vi "PIDAutoTune_OpenLoop_ChooseMethod.vi"(4 "Sampling Time dt (s)":dbl, 5 "Constant Type":T2(ring), 6 "Kn":dbl, 7 "Type of Controller":u16(ring) items=["P", "PI", "PID"], 8 "Tune":bool, 9 "CO Offset":dbl=0.25, 10 "Measurement  (PV)":dbl, 11 "Control Output (Co)":dbl) -> (0 "Plant and Test Data":T3, 1 "New Tuning Parameters":T1, 2 "Tuning Done":bool, 3 "Adj CO":dbl)   [LabVIEW 2019, in "Trajectory_Library.lvlib"]
uses:
  Timer_New.vi
  LinearFilter_ResetToValue.vi
  LinearFilter_Calculate.vi
  <vilib>/Utility/semaphor.llb/Obtain Semaphore Reference.vi
  Timer_Reset.vi
  Timer_Start.vi
  Timer_Stop.vi
  Timer_HasPeriodPassedOnce.vi
  <vilib>/addons/control/pid/autopid.llb/PID Autotuning Design (Auto).vi
  <vilib>/addons/control/pid/autopid.llb/PID Autotuning Design (Chien-Hrones-Reswick).vi
  <vilib>/Analysis/Matrix/Numeric/Conversions/Array To Matrix - RA.vi
  LinearFilter_MovingAverage.vi
  LinearFilter_LowPassBW1.vi
  LinearFilter_LowPassBW2.vi
  LinearFilter_HighPassBW1.vi
  LinearFilter_HighPassBW2.vi
  Trajectory_Library.lvlib
  <vilib>/addons/control/pid/NI_PID_autopid.lvlib
  <vilib>/ptbypt/NI_PtbyPt.lvlib
  <vilib>/Analysis/Matrix/NI_Matrix.lvlib
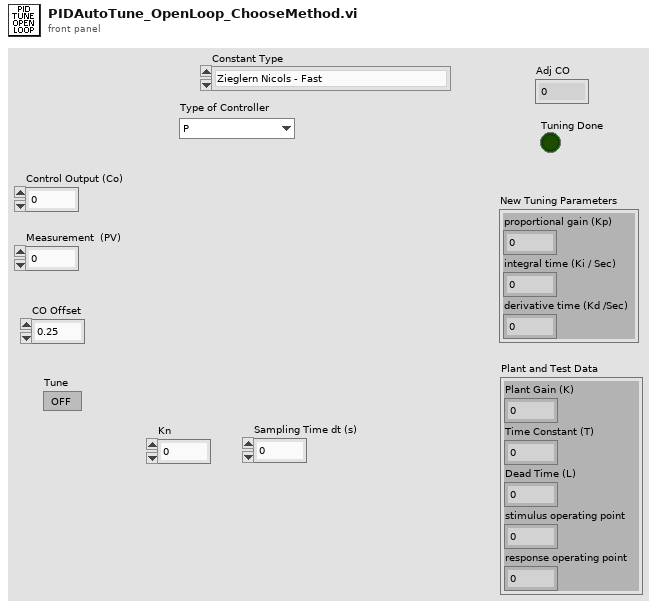
[diagram p1: front panel]
types:
  T1 = cluster{"proportional gain (Kp)":dbl, "integral time (Ki / Sec)":dbl, "derivative time (Kd /Sec)":dbl}
  T2 = enum16{"Zieglern Nicols - Fast", "Ziegler Nicols - Normal", "Ziegler Nicols - Slow", "CHR regulator - 0% overshoot", "CHR regulator - 20% overshoot", "CHR servo - 0 % overshoot", "CHR servo - 20% overshoot"}
  T3 = cluster{"Plant Gain (K)":dbl, "Time Constant (T)":dbl, "Dead Time (L)":dbl, "stimulus operating point":dbl, "response operating point":dbl}
  T4 = enum16{"Moving Average", "Low Pass 1st Order Butterworth", "Low Pass 2nd Order Butterworth", "High Pass 1st Order Butterworth", "High Pass 2nd Order Butterworth"}
  T5 = cluster{"proportional gain (Kc)":dbl, "integral time (Ti, min)":dbl, "derivative time (Td, min)":dbl}
  T6 = cluster{"Plant Gain (K)":dbl, "Time Constant (T)":dbl, "Dead Time (L)":dbl}
  T7 = typedef "NI_Matrix.lvlib/RealMatrix.ctl" = dbl[][]
  T8 = cluster{"Plant Gain (K)":dbl, "Time Constant (T)":dbl, "Dead Time (L)":dbl, "stimulus offset":dbl, "response offset":dbl}
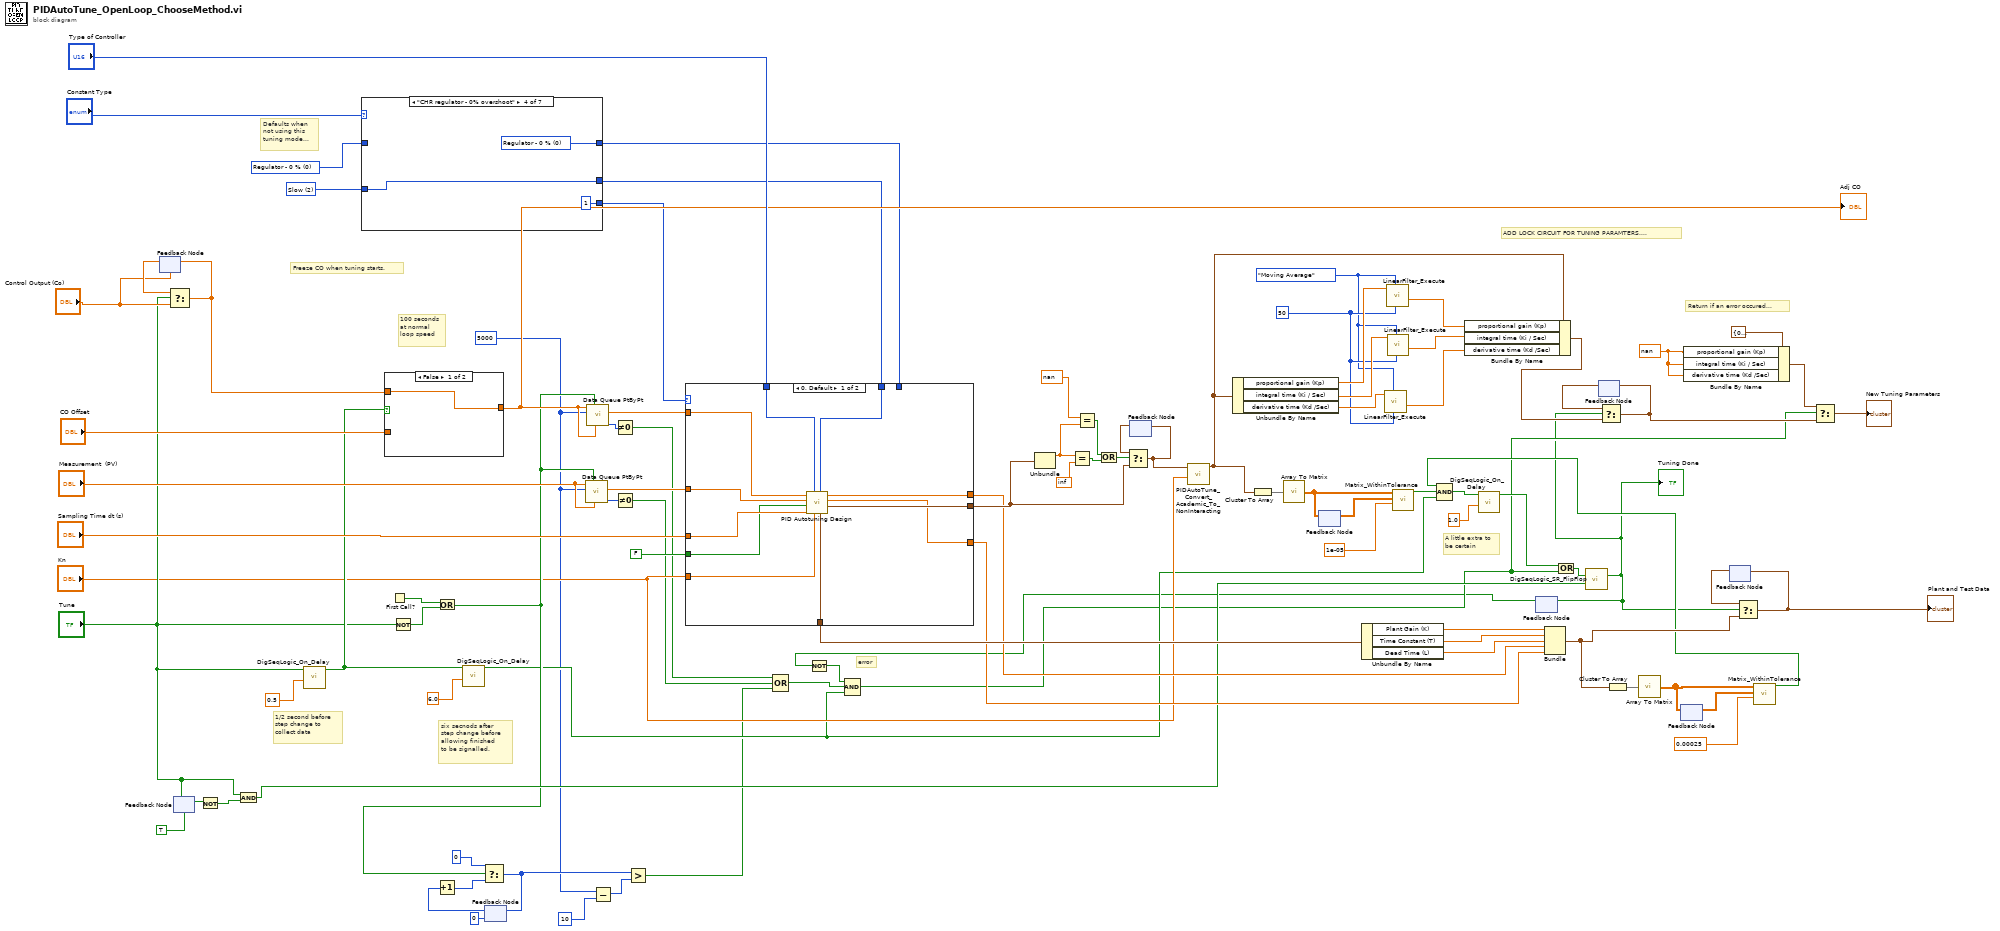
[diagram p0: block diagram]
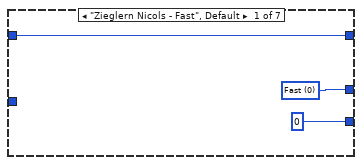
[diagram p2: hidden frame]
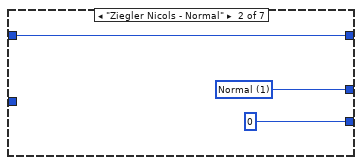
[diagram p3: hidden frame]
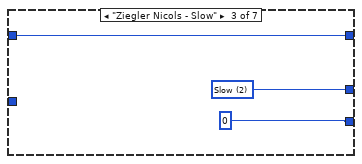
[diagram p4: hidden frame]
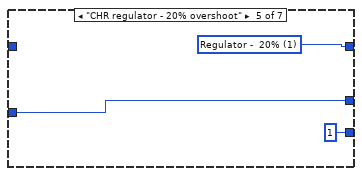
[diagram p5: hidden frame]
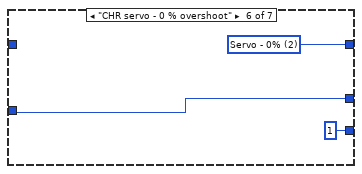
[diagram p6: hidden frame]
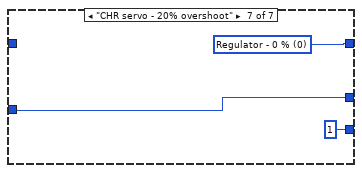
[diagram p7: hidden frame]
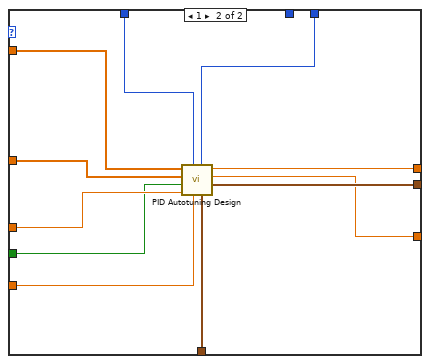
[diagram p8: hidden frame]
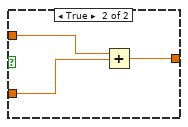
[diagram p9: hidden frame]
diagram:
  w22 = nan
  w50 = 50 ("Samples")
  w49 = T4."Moving Average" ("Filter Type")
  w55 = u16 2 items=["Fast", "Normal", "Slow"] ("Ziegler-Nichols Speed")
  w56 = u16 0 items=["Regulator - 0 %", "Regulator -  20%", "Servo - 0%", "Servo - 20%"] ("Tuning specifications")
  w8 = 5000 ("sample length")
  # "error"
  # "Return if an error occured..."
  # "A little extra to\nbe certain"
  # "Defaults when\nnot using this\ntuning mode..."
  # "100 seconds\nat normal\nloop speed"
  # "Freeze CO when tuning starts."
  # "ADD LOCK CIRCUIT FOR TUNING PARAMTERS...."
  # "six secnods after\nstep change before\nallowing finished \nto be signalled."
  # "1/2 second before\nstep change to\ncollect data"
  n1 = feedback #1("Control Output (Co)") -> (w73:dbl)
  n2 = Select(t=w73, s="Tune", f="Control Output (Co)") -> (s? t:f=w74:dbl)
  n3 = feedback-in #1(w74) -> ()
  n4 = feedback-in #2("Tune") -> ()
  n5 = feedback #2(TRUE ("Tune")) -> (w69:bool)
  n6 = Not(x=w69) -> (.not. x?=w67:bool)
  n7 = And(x="Tune", y=w67) -> (x .and. y?=w66:bool)
  n8 = call "DigSeqLogic_On_Delay.vi"("Delay"=0.5, "Input"="Tune") -> ("Output"=w76:bool)  [unwired: 8 in, 1 out]
  n9 = case shown="\"CHR regulator - 0% overshoot\"" "Constant Type" {
    tunnel: [w99 w102 w105 w106 w109 w112 w115] -> w59
    tunnel: [0 0 0 1 1 1 1] -> w58
    tunnel: [w97 w100 w103 w107 w110 w113 w116] -> w57
    tunnel: w56 -> [w97 w100 w103 _ _ _ _]
    tunnel: w55 -> [_ _ _ w106 w109 w112 w115]
    frame "Zieglern Nicols - Fast", Default {
      w99 = u16 0 items=["Fast", "Normal", "Slow"] ("Ziegler-Nichols Speed")
    }
    frame "Ziegler Nicols - Normal" {
      w102 = u16 1 items=["Fast", "Normal", "Slow"] ("Ziegler-Nichols Speed")
    }
    frame "Ziegler Nicols - Slow" {
      w105 = u16 2 items=["Fast", "Normal", "Slow"] ("Ziegler-Nichols Speed")
    }
    frame "CHR regulator - 0% overshoot" {
      w107 = u16 0 items=["Regulator - 0 %", "Regulator -  20%", "Servo - 0%", "Servo - 20%"] ("Tuning specifications")
    }
    frame "CHR regulator - 20% overshoot" {
      w110 = u16 1 items=["Regulator - 0 %", "Regulator -  20%", "Servo - 0%", "Servo - 20%"] ("Tuning specifications")
    }
    frame "CHR servo - 0 % overshoot" {
      w113 = u16 2 items=["Regulator - 0 %", "Regulator -  20%", "Servo - 0%", "Servo - 20%"] ("Tuning specifications")
    }
    frame "CHR servo - 20% overshoot" {
      w116 = u16 0 items=["Regulator - 0 %", "Regulator -  20%", "Servo - 0%", "Servo - 20%"] ("Tuning specifications")
    }
  }
  n10 = case shown="False" w76 {
    tunnel: w74 -> [w118 w121]
    tunnel: "CO Offset" -> [_ w120]
    tunnel: [w118 w119] -> w71
    frame False {
    }
    frame True {
      n11 = Add(x=w121, y=w120) -> (x+y=w119:dbl)
    }
  }
  "Adj CO" <- w71
  n12 = First Call?() -> (First Call?: T/F=w21:bool)
  n13 = Not(x="Tune") -> (.not. x?=w20:bool)
  n14 = Or(x=w21, y=w20) -> (x .or. y?=w18:bool)
  n15 = call "DigSeqLogic_On_Delay.vi"("Delay"=6.0, "Input"=w76) -> ("Output"=w15:bool)  [unwired: 8 in, 1 out]
  n16 = feedback #3(0) -> (w12:i32)
  n17 = Increment(x=w12) -> (x+1=w11:i32)
  n18 = Select(t=0, s=w18, f=w11) -> (s? t:f=w10:i32)
  n19 = feedback-in #3(w10) -> ()
  n20 = call <vilib>:"Data Queue PtByPt.vi"("initial queue element"="Measurement  (PV)", "initialize"=w18, "sample length"=w8, "input data point"="Measurement  (PV)") -> ("error"=w29:i32, "Current Queue"=w90:dbl[])  [unwired: 3 in, 3 out]
  n21 = call <vilib>:"Data Queue PtByPt.vi"("initial queue element"=w71, "initialize"=w18, "sample length"=w8, "input data point"=w71) -> ("error"=w30:i32, "Current Queue"=w91:dbl[])  [unwired: 3 in, 3 out]
  n22 = Subtract(x=w8, y=10) -> (x-y=w9:i32)
  n23 = Not Equal To 0?(x=w30) -> (x != 0?=w5:bool)
  n24 = Not Equal To 0?(x=w29) -> (x != 0?=w4:bool)
  n25 = Greater?(x=w10, y=w9) -> (0:w6:bool)
  n26 = case shown="0, Default" w58 {
    tunnel: [w132 w143] -> w95
    tunnel: "Sampling Time dt (s)" -> [w131 w142]
    tunnel: w91 -> [w130 w141]
    tunnel: w90 -> [w129 w140]
    tunnel: "Type of Controller" -> [w128 w139]
    tunnel: [w127 w138] -> w85
    tunnel: [w126 w137] -> w81
    tunnel: [w125 w136] -> w80
    tunnel: "Kn" -> [w124 w135]
    tunnel: w59 -> [w123 _]
    tunnel: w57 -> [_ w134]
    tunnel: FALSE ("closed-loop?") -> [w122 w133]
    frame 0, Default {
      n27 = call-poly <vilib>:"PID Autotuning Design.vi"("Ziegler-Nichols Speed"=w123, "Controller Gain (K)"=w124, "Type of Controller"=w128, "dt (s)"=w131, "closed-loop?"=w122, "Response signal"=w129, "Stimulus signal"=w130) -> ("PID gains"=w132:T5, "response operating point"=w125:dbl, "stimulus operating point"=w126:dbl, "Plant Parameters"=w127:T6)  [unwired: 1 in]
    }
    frame 1 {
      n28 = call-poly <vilib>:"PID Autotuning Design.vi"("Tuning specifications"=w134, "Controller Gain (K)"=w135, "Type of Controller"=w139, "dt (s)"=w142, "closed-loop?"=w133, "Response signal"=w140, "Stimulus signal"=w141) -> ("PID gains"=w143:T5, "response offset"=w136:dbl, "stimulus offset"=w137:dbl, "Plant Parameters"=w138:T6)  [unwired: 1 in]
    }
  }
  n29 = Compound Arithmetic op=OR(w5, w4, w6) -> (w17:bool)
  n30 = Unbundle(w95) -> ("proportional gain (Kc)"=w41:dbl)  [unwired: 2 out]
  n31 = Equal?(x=w41, y=inf) -> (x = y?=w38:bool)
  n32 = Equal?(x=nan, y=w41) -> (x = y?=w39:bool)
  n33 = Or(x=w39, y=w38) -> (x .or. y?=w40:bool)
  n34 = feedback #4() -> (w94:T5)  [unwired: 1 in]
  n35 = Select(t=w94, s=w40, f=w95) -> (s? t:f=w96:T5)
  n36 = feedback-in #4(w96) -> ()
  n37 = call "PIDAutoTune_Convert_Academic_To_NonInteracting.vi"("Kn"="Kn", "PID gains NI Academic"=w96) -> ("PID Gains Non Interacting"=w37:T1)  [unwired: 9 in]
  n38 = Unbundle By Name(w37) -> ("proportional gain (Kp)"=w51:dbl, "integral time (Ki / Sec)"=w52:dbl, "derivative time (Kd /Sec)"=w53:dbl)
  n39 = Cluster To Array(cluster=w37) -> (array=w87:dbl[])
  n40 = call-poly <vilib>:"Array To Matrix.vi"("Real 1D Array"=w87) -> ("Real Matrix (Column Vector)"=w44:T7)
  n41 = feedback-in #5(w44) -> ()
  n42 = feedback #5() -> (w43:T7)  [unwired: 1 in]
  n43 = Unbundle By Name(w85) -> ("Plant Gain (K)"=w84:dbl, "Time Constant (T)"=w83:dbl, "Dead Time (L)"=w82:dbl)
  n44 = call "LinearFilter_Execute.vi"("Samples"=w50, "Filter Type"=w49, "Input"=w53) -> ("Output"=w46:dbl)  [unwired: 7 in, 1 out]
  n45 = call "LinearFilter_Execute.vi"("Samples"=w50, "Filter Type"=w49, "Input"=w51) -> ("Output"=w48:dbl)  [unwired: 7 in, 1 out]
  n46 = call "LinearFilter_Execute.vi"("Samples"=w50, "Filter Type"=w49, "Input"=w52) -> ("Output"=w47:dbl)  [unwired: 7 in, 1 out]
  n47 = call "Matrix_WithinTolerance.vi"("Tolerance"=1e-05, "Matrix B"=w43, "Matrix A"=w44) -> ("WithinTolerance"=w75:bool)  [unwired: 7 in, 1 out]
  n48 = Bundle By Name(cluster=w37, "proportional gain (Kp)"=w48, "integral time (Ki / Sec)"=w47, "derivative time (Kd /Sec)"=w46) -> (w45:T1)
  n49 = feedback #6() -> (w1:bool)  [unwired: 1 in]
  n50 = Not(x=w1) -> (.not. x?=w3:bool)
  n51 = Compound Arithmetic op=AND(w3, w17, w15) -> (w14:bool)
  n52 = Bundle("Plant Gain (K)"=w84, "Time Constant (T)"=w83, "Dead Time (L)"=w82, "stimulus offset"=w81, "response offset"=w80) -> (w35:T8)  [unwired: 1 in]
  n53 = feedback #7() -> (w63:T1)  [unwired: 1 in]
  n54 = Cluster To Array(cluster=w35) -> (array=w36:dbl[])
  n55 = call-poly <vilib>:"Array To Matrix.vi"("Real 1D Array"=w36) -> ("Real Matrix (Column Vector)"=w32:T7)
  n56 = feedback #8() -> (w33:T7)  [unwired: 1 in]
  n57 = feedback-in #8(w32) -> ()
  n58 = Bundle By Name(cluster=T1 {"proportional gain (Kp)"=0.0, "integral time (Ki / Sec)"=0.0, "derivative time (Kd /Sec)"=0.0} ("t"), "proportional gain (Kp)"=w22, "integral time (Ki / Sec)"=w22, "derivative time (Kd /Sec)"=w22) -> (w23:T1)
  n59 = feedback #9() -> (w64:T8)  [unwired: 1 in]
  n60 = call "Matrix_WithinTolerance.vi"("Tolerance"=0.00025, "Matrix B"=w33, "Matrix A"=w32) -> ("WithinTolerance"=w31:bool)  [unwired: 7 in, 1 out]
  n61 = Compound Arithmetic op=AND(w31, w75, w15) -> (w62:bool)
  n62 = call "DigSeqLogic_On_Delay.vi"("Delay"=1.0, "Input"=w62) -> ("Output"=w27:bool)  [unwired: 8 in, 1 out]
  n63 = Or(x=w27, y=w14) -> (x .or. y?=w28:bool)
  n64 = call "DigSeqLogic_SR_FlipFlop.vi"("Set"=w28, "Reset"=w66) -> ("Output"=w2:bool)  [unwired: 12 in, 1 out]
  "Tuning Done" <- w2
  n65 = feedback-in #6(w2) -> ()
  n66 = Select(t=w63, s=w2, f=w45) -> (s? t:f=w25:T1)
  n67 = feedback-in #7(w25) -> ()
  n68 = Select(t=w64, s=w2, f=w35) -> (s? t:f=w65:T8)
  "Plant and Test Data" <- w65
  n69 = feedback-in #9(w65) -> ()
  n70 = Select(t=w23, s=w14, f=w25) -> (s? t:f=→"New Tuning Parameters":T1)
